vi "Write G08 Settings.vi"(8 "error in (no error)":errorcluster, 10 "G08Settings":T1={"Gate Terminate"=TRUE, "Gate Level"=1.0, "Gate Delay (µs)"=0.0, "Step Back Time (µs)"=0.0, "Burst Counter"=0} {"Step Back Time (µs)" min=0.0 format="%.6f"; "Gate Delay (µs)" format="%.3f"; "Gate Level" min=-2.5 max=2.5 format="%.3g"}, 11 "BME_DG_G08 in":refnum<class "BME_DG_G08.lvclass">) -> (0 "error out":errorcluster, 3 "BME_DG_G08 out":refnum<class "BME_DG_G08.lvclass">)   [LabVIEW 2009, in "BME_DG_G08.lvclass"]
uses:
  BME_DG_G08.lvclass
  G08TriggerSettings.ctl
  BME_DG_G08.lvclass/BME_DG_G08.ctl
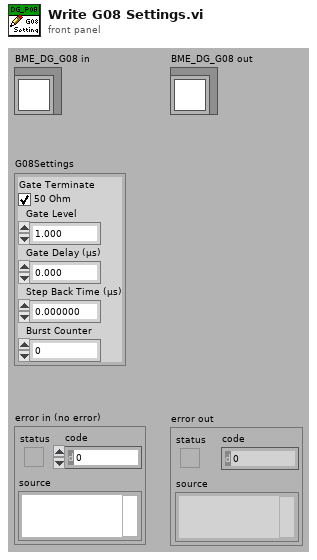
[diagram p1: front panel]
types:
  T1 = typedef "BME_DG_G08.lvclass/G08TriggerSettings.ctl" = cluster{"Gate Terminate":bool, "Gate Level":dbl, "Gate Delay (µs)":dbl, "Step Back Time (µs)":dbl, "Burst Counter":u32}
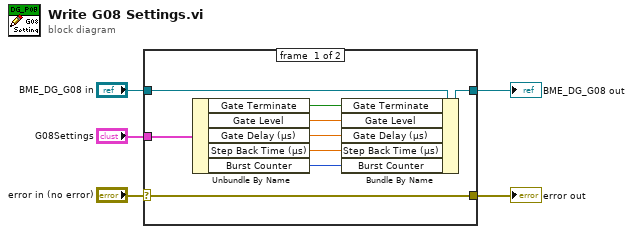
[diagram p0: block diagram]
diagram:
  n1 = case shown="No Error" "error in (no error)" {
    selector: "error in (no error)" -> [w6 w16]
    tunnel: [w6 w16] -> w5
    tunnel: [w14 w15] -> w4
    tunnel: "BME_DG_G08 in" -> [w7 w15]
    tunnel: "G08Settings" -> [w8 _]
    frame #0 {
      n2 = Unbundle By Name(w8) -> ("Gate Terminate"=w13:bool, "Gate Level"=w12:dbl, "Gate Delay (µs)"=w11:dbl, "Step Back Time (µs)"=w10:dbl, "Burst Counter"=w9:u32)
      n3 = Bundle By Name(cluster=w7, "Gate Terminate"=w13, "Gate Level"=w12, "Gate Delay (µs)"=w11, "Step Back Time (µs)"=w10, "Burst Counter"=w9) -> (w14:refnum<class "BME_DG_G08.lvclass">)
    }
    frame #1 {
    }
  }
  "error out" <- w5
  "BME_DG_G08 out" <- w4
